vi "SubVI_SVM_gridsearch_n_fold.vi"(0 "Max Passes":i32=15, 5 "Training Labels":dbl[][](array[numeric]), 7 "Training Data":dbl[][](array[numeric]), 9 "Array":string[](array[string]), 10 "Optimizer\nMetric":string="F1", 11 "C":dbl[](array[numeric]), 12 "Gamma":dbl[](array[numeric])) -> (1 "Performance":T2, 2 "Hyperparameters":T1, 4 "Kernel Type":string, 6 "Alpha (idx)":dbl[][](array[numeric]), 8 "w":dbl[][](array[numeric]), 13 "label (idx)":dbl[][](array[numeric]), 14 "Training (idx)":dbl[][](array[numeric]), 15 "b":dbl)   [LabVIEW 2020]
uses:
  <vilib>/Analysis/baseanly.llb/Mean (DBL).vi
  <vilib>/Analysis/1siggen.llb/Riffle Array (DBL).vi
  <vilib>/Analysis/NI_AALBase.lvlib
panel:
  out "Numeric 3":i32
  out "Numeric 2":i32
  out "Numeric":i32
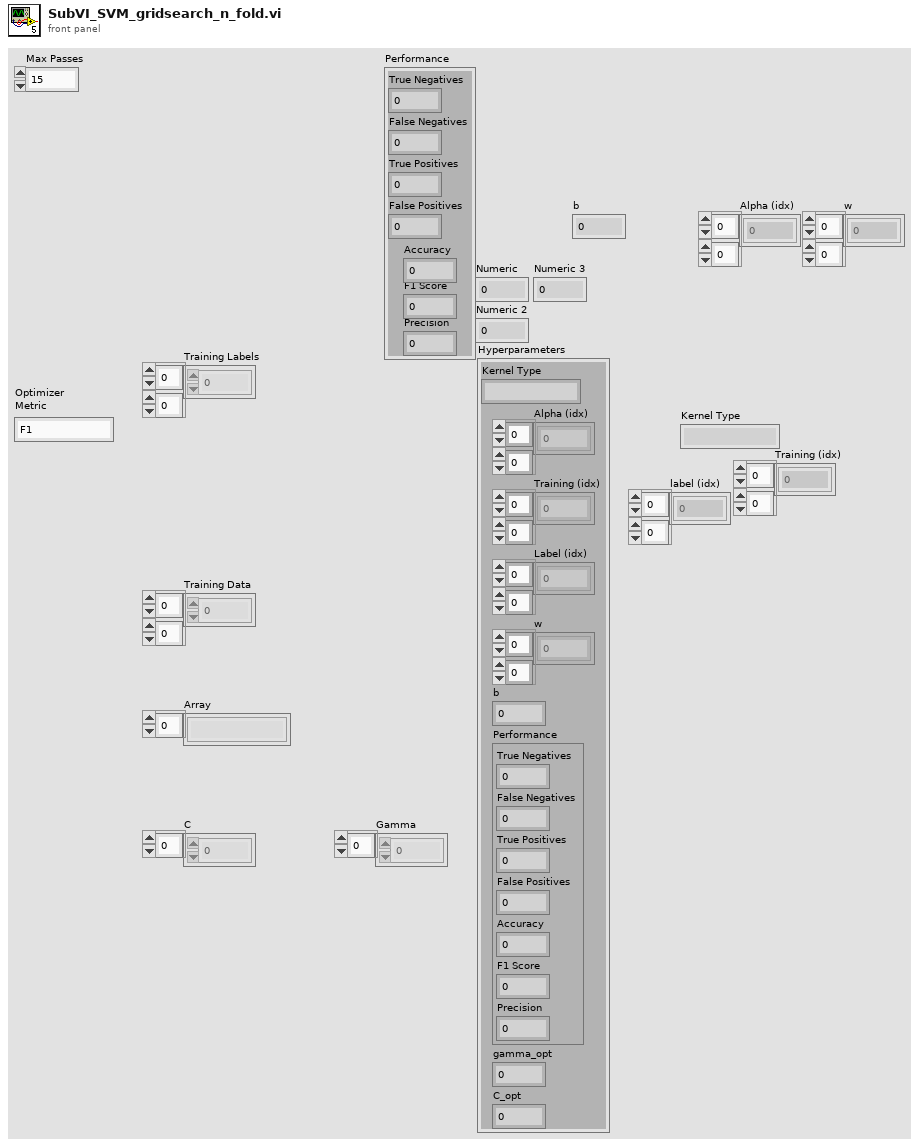
[diagram p1: front panel]
types:
  T1 = cluster{"Kernel Type":string, "Alpha (idx)":dbl[][], "Training (idx)":dbl[][], "Label (idx)":dbl[][], "w":dbl[][], "b":dbl, "Performance":cluster{"True Negatives":i32, "False Negatives":i32, "True Positives":i32, "False Positives":i32, "Accuracy":dbl, "F1 Score":dbl, "Precision":dbl}, "gamma_opt":dbl, "C_opt":dbl}
  T2 = cluster{"True Negatives":i32, "False Negatives":i32, "True Positives":i32, "False Positives":i32, "Accuracy":dbl, "F1 Score":dbl, "Precision":dbl}
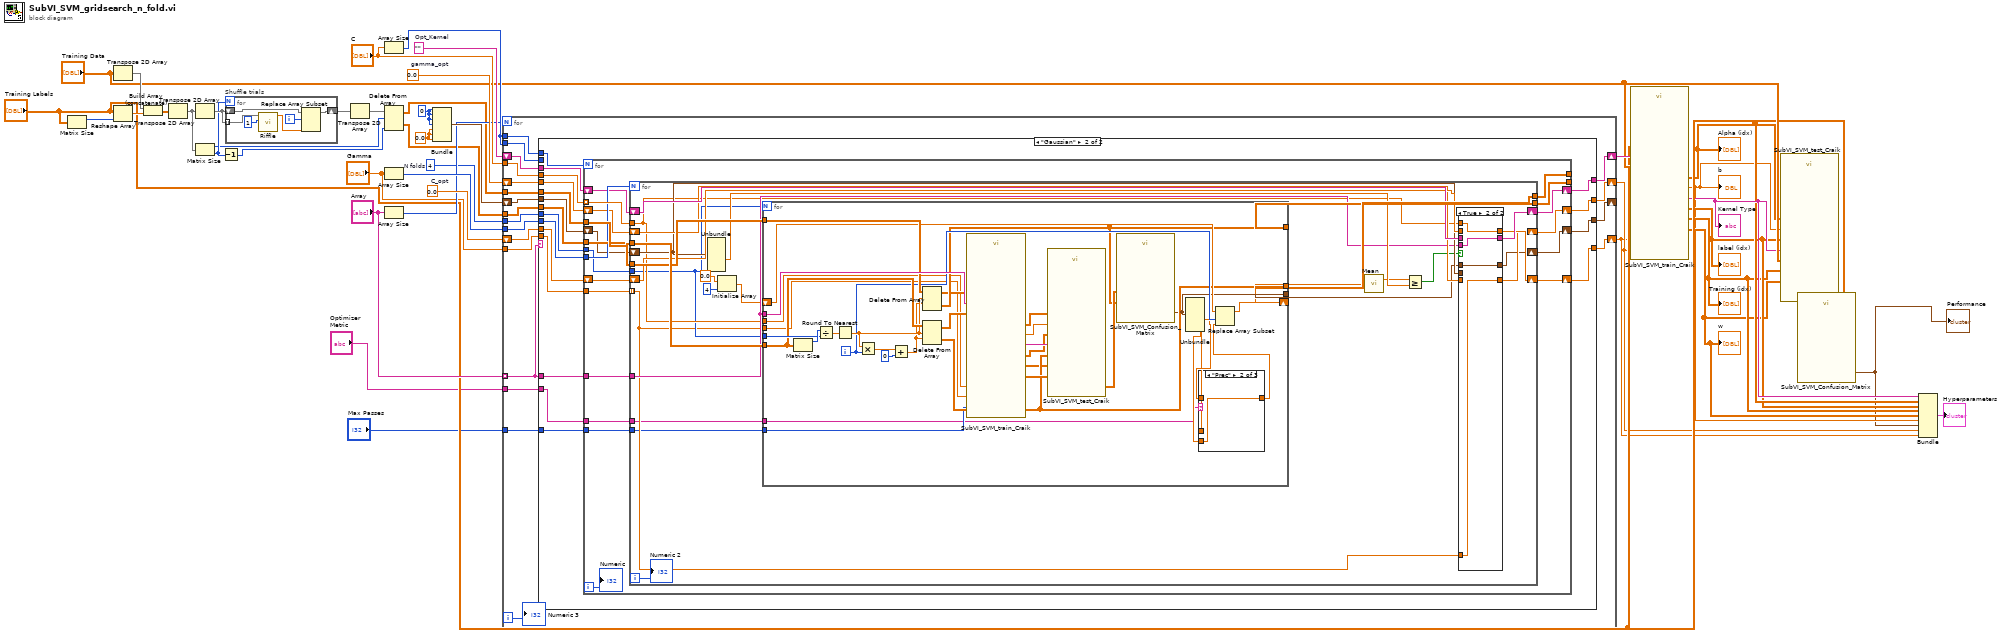
[diagram p0: block diagram]
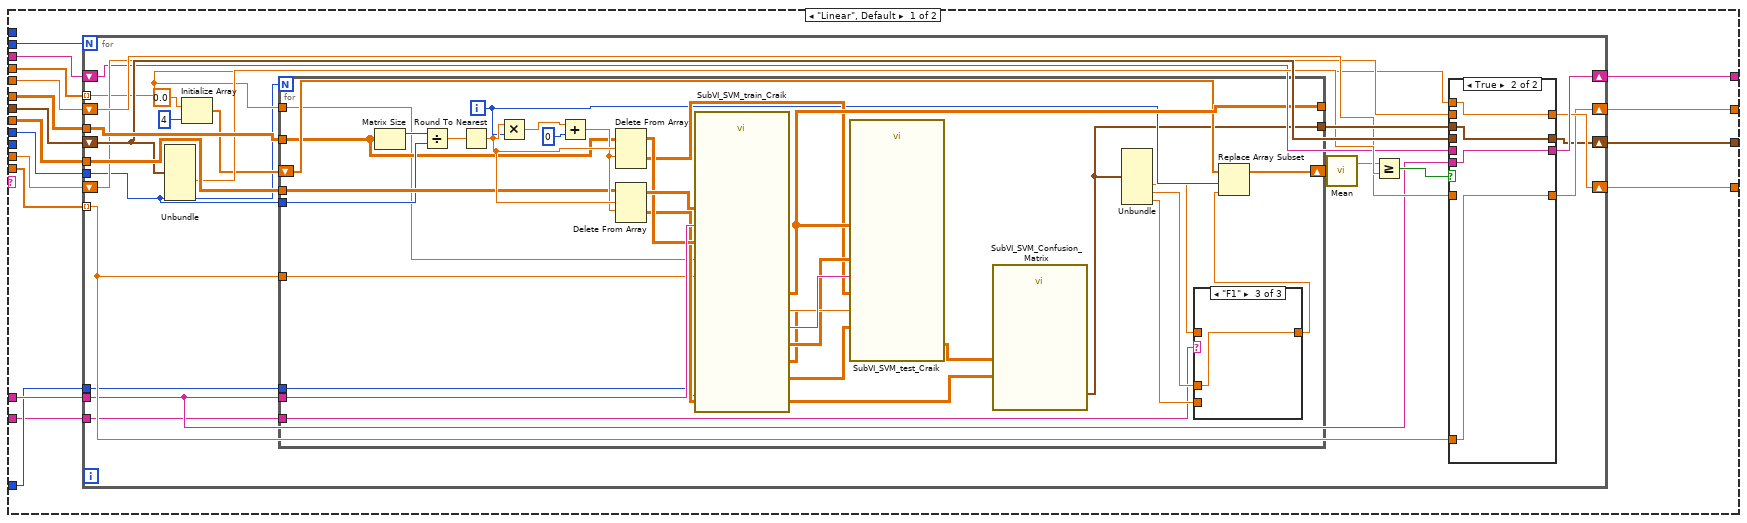
[diagram p2: hidden frame]
diagram:
  w32 = 4  # N folds
  w3 = 0.0
  w38 = 0
  w35 = ""  # Opt_Kernel
  w37 = 0.0  # gamma_opt
  w36 = 0.0  # C_opt
  n1 = Matrix Size(0:"Training Labels") -> (1:w29:i32)  [unwired: 1 out]
  n2 = Transpose 2D Array(2D array="Training Data") -> (transposed array=w28:dbl[][])
  n3 = Reshape Array("Training Labels", w29) -> (w31:dbl[])
  n4 = Build Array (concatenate)(w28, w31) -> (w30:dbl[][])
  n5 = Transpose 2D Array(2D array=w30) -> (transposed array=w21:dbl[][])
  n6 = Transpose 2D Array(2D array=w21) -> (transposed array=w27:dbl[][])
  n7 = Matrix Size(0:w21) -> (1:w23:i32, 2:w24:i32)
  n8 = Decrement(x=w24) -> (x-1=w22:i32)
  n9 = for "Shuffle trials" {
    N: w24 -> [_]
    tunnel: w27 -> [w48] mode=indexing
    shift-right: [w43] -> w26
    shift-left: w27 -> [w46]
    i -> [w44]
    n10 = call-poly <vilib>:"Riffle.vi"("seed"=1, "X"=w48) -> ("Riffled {X}"=w45:dbl[])  [unwired: 7 in, 2 out]
    n11 = Replace Array Subset(array=w46, new element=w45, index (row)=w44) -> (w43:dbl[][])  [unwired: 1 in]
  }
  n12 = Transpose 2D Array(2D array=w26) -> (transposed array=w25:dbl[][])
  n13 = Array Size(array="C") -> (size(s)=w40:i32)
  n14 = Delete From Array(array=w25, length=w23, index (col)=w22) -> (deleted portion=w19:dbl[][], array with subset deleted=w20:dbl[][])  [unwired: 1 in]
  n15 = Array Size(array="Gamma") -> (size(s)=w41:i32)
  n16 = Array Size(array="Array") -> (size(s)=w34:i32)
  n17 = Bundle(w38, w38, w38, w38, w3, w3, w3) -> (w39:cluster{i32, i32, i32, i32, dbl, dbl, dbl})  [unwired: 1 in]
  n18 = for {
    N: w34 -> [_]
    tunnel: "C" -> [w68]
    tunnel: "Array" -> [w64] mode=indexing
    tunnel: w20 -> [w67]
    tunnel: w19 -> [w66]
    tunnel: "Gamma" -> [w65]
    tunnel: w40 -> [w63]
    shift-right: [w61] -> w18
    shift-left: w35 -> [w62]
    shift-right: [w59] -> w6
    shift-left: w36 -> [w60]
    shift-right: [w57] -> w7
    shift-left: w37 -> [w58]
    shift-right: [w55] -> _
    shift-left: w39 -> [w56]
    tunnel: w40 -> [w54]
    tunnel: w41 -> [w53]
    tunnel: w32 -> [w52]
    tunnel: "Max Passes" -> [w50]
    tunnel: "Optimizer\nMetric" -> [w49]
    i -> [w51]
    n19 = case shown="\"Gaussian\"" w64 {
      tunnel: w68 -> [w85 w171]
      tunnel: w64 -> [w84 w170]
      tunnel: w67 -> [w83 w169]
      tunnel: w66 -> [w82 w168]
      tunnel: w65 -> [w81 w157]
      tunnel: w63 -> [w80 _]
      tunnel: w62 -> [w79 w165]
      tunnel: [w78 w158] -> w61
      tunnel: w60 -> [w77 w164]
      tunnel: [w76 w159] -> w59
      tunnel: w58 -> [w75 w163]
      tunnel: [w74 w160] -> w57
      tunnel: w56 -> [w73 w162]
      tunnel: [w72 w161] -> w55
      tunnel: w54 -> [_ w167]
      tunnel: w53 -> [_ w166]
      tunnel: w52 -> [w71 w156]
      tunnel: w50 -> [w70 w155]
      tunnel: w49 -> [w69 w154]
      frame "Linear", Default {
        n20 = for {
          N: w80 -> [_]
          tunnel: w85 -> [w94] mode=indexing
          tunnel: w84 -> [w99]
          tunnel: w83 -> [w109]
          tunnel: w82 -> [w108]
          tunnel: w81 -> [w102] mode=indexing
          shift-right: [w98] -> w78
          shift-left: w79 -> [w100]
          shift-right: [w97] -> w76
          shift-left: w77 -> [w101]
          shift-right: [w96] -> w74
          shift-left: w75 -> [w103]
          shift-right: [w95] -> w72
          shift-left: w73 -> [w107]
          tunnel: w71 -> [w88]
          tunnel: w70 -> [w87]
          tunnel: w69 -> [w86]
          n21 = Unbundle(w107) -> (w105:dbl)  [unwired: 6 out]
          n22 = Initialize Array(0.0 ("element"), 4 ("dimension size")) -> (w91:dbl[])
          n23 = for {
            N: w88 -> [_]
            tunnel: w109 -> [w119]
            tunnel: w108 -> [w128]
            tunnel: [w138] -> _
            tunnel: [w115] -> w106
            tunnel: w102 -> [w118]
            tunnel: w99 -> [w135]
            tunnel: w94 -> [w117]
            shift-right: [w121] -> w90
            shift-left: w91 -> [w123]
            tunnel: w88 -> [w120]
            tunnel: w87 -> [w116]
            tunnel: w86 -> [w110]
            i -> [w122]
            n24 = Matrix Size(0:w119) -> (1:w134:i32)  [unwired: 1 out]
            n25 = Divide(x=w134, y=w120) -> (x/y=w133:dbl)
            n26 = Round To Nearest(number=w133) -> (nearest integer value=w130:dbl)
            n27 = Multiply(x=w130, y=w122) -> (x*y=w131:dbl)
            n28 = Add(x=w131, y=0) -> (x+y=w129:dbl)
            n29 = Delete From Array(array=w119, length=w130, index (row)=w129) -> (deleted portion=w125:dbl[][], array with subset deleted=w126:dbl[][])  [unwired: 1 in]
            n30 = Delete From Array(array=w128, length=w130, index (row)=w129) -> (deleted portion=w124:dbl[][], array with subset deleted=w127:dbl[][])  [unwired: 1 in]
            n31 = call "SubVI_SVM_train_Craik.vi"("Max Passes"=w116, "C"=w117, "Label Data"=w127, "Gamma"=w118, "Linear or Gaussian"=w135, "Training Data"=w126) -> ("Alpha (idx)"=w138:dbl[][], "Label (idx)"=w136:dbl[][], "b"=w139:dbl, "Training (idx)"=w137:dbl[][], "w"=w140:dbl[][], "Kernel Type"=w141:string)
            n32 = call "SubVI_SVM_test_Craik.vi"("Alpha (idx)"=w138, "Testing Data"=w125, "Label (idx)"=w136, "training (idx)"=w137, "Linear or Gaussian"=w141, "b"=w139, "w"=w140) -> ("Prediction"=w142:dbl[][])  [unwired: 4 in]
            n33 = call "SubVI_SVM_Confusion_Matrix.vi"("Real Labels"=w124, "Predictions"=w142) -> ("Performance"=w115:T2)  [unwired: 9 in]
            n34 = Unbundle(w115) -> ("Accuracy"=w112:dbl, "F1 Score"=w113:dbl, "Precision"=w114:dbl)  [unwired: 4 out]
            n35 = case shown="\"F1\"" w110 {
              tunnel: w114 -> [_ w144 _]
              tunnel: w113 -> [_ _ w145]
              tunnel: w112 -> [w143 _ _]
              tunnel: [w143 w144 w145] -> w111
              frame "Acc", Default {
              }
              frame "Prec" {
              }
              frame "F1" {
              }
            }
            n36 = Replace Array Subset(array=w123, new element=w111, index=w122) -> (w121:dbl[])
          }
          n37 = call-poly <vilib>:"Mean.vi"("X"=w90) -> ("mean"=w89:dbl)  [unwired: 1 out]
          n38 = Greater Or Equal?(x=w89, y=w105) -> (x >= y?=w104:bool)
          n39 = case shown="True" w104 {
            tunnel: w107 -> [w146 _]
            tunnel: w106 -> [_ w150]
            tunnel: w103 -> [w147 _]
            tunnel: w102 -> [_ w151]
            tunnel: w94 -> [_ w152]
            tunnel: w101 -> [w148 _]
            tunnel: w100 -> [w149 _]
            tunnel: w99 -> [_ w153]
            tunnel: [w149 w153] -> w98
            tunnel: [w148 w152] -> w97
            tunnel: [w147 w151] -> w96
            tunnel: [w146 w150] -> w95
            frame False {
            }
            frame True {
            }
          }
        }
      }
      frame "Gaussian" {
        n40 = for {
          N: w167 -> [_]
          tunnel: w171 -> [w191] mode=indexing
          tunnel: [w190] -> _
          tunnel: [w189] -> _
          tunnel: w170 -> [w188]
          tunnel: w169 -> [w187]
          tunnel: w168 -> [w186]
          tunnel: w157 -> [w185]
          tunnel: w166 -> [w184]
          shift-right: [w179] -> w158
          shift-left: w165 -> [w183]
          shift-right: [w178] -> w159
          shift-left: w164 -> [w182]
          shift-right: [w177] -> w160
          shift-left: w163 -> [w181]
          shift-right: [w176] -> w161
          shift-left: w162 -> [w180]
          tunnel: w156 -> [w175]
          tunnel: w155 -> [w173]
          tunnel: w154 -> [w172]
          i -> [w174]
          n41 = for {
            N: w184 -> [_]
            tunnel: w191 -> [w207]
            tunnel: [w218] -> w190
            tunnel: [w217] -> w189
            tunnel: w188 -> [w208]
            tunnel: w187 -> [w216]
            tunnel: w186 -> [w215]
            tunnel: w185 -> [w196] mode=indexing
            shift-right: [w205] -> w179
            shift-left: w183 -> [w214]
            shift-right: [w204] -> w178
            shift-left: w182 -> [w213]
            shift-right: [w203] -> w177
            shift-left: w181 -> [w212]
            shift-right: [w193] -> w176
            shift-left: w180 -> [w210]
            tunnel: w175 -> [w202]
            tunnel: w173 -> [w194]
            tunnel: w172 -> [w192]
            i -> [w195]
            n42 = Unbundle(w210) -> (w211:dbl)  [unwired: 6 out]
            n43 = Initialize Array(0.0 ("element"), 4 ("dimension size")) -> (w199:dbl[])
            n44 = for {
              N: w202 -> [_]
              tunnel: [w231] -> w218
              tunnel: [w233] -> w217
              tunnel: w216 -> [w240]
              tunnel: w215 -> [w239]
              tunnel: w208 -> [w249]
              tunnel: w207 -> [w228]
              tunnel: w196 -> [w229]
              tunnel: [w224] -> w206
              tunnel: w202 -> [w244]
              shift-right: [w234] -> w198
              shift-left: w199 -> [w236]
              tunnel: w194 -> [w225]
              tunnel: w192 -> [w219]
              i -> [w235]
              n45 = Matrix Size(0:w240) -> (1:w245:i32)  [unwired: 1 out]
              n46 = Divide(x=w245, y=w244) -> (x/y=w243:dbl)
              n47 = Round To Nearest(number=w243) -> (nearest integer value=w238:dbl)
              n48 = Multiply(x=w238, y=w235) -> (x*y=w241:dbl)
              n49 = Add(x=w241, y=0) -> (x+y=w237:dbl)
              n50 = Delete From Array(array=w239, length=w238, index (row)=w237) -> (deleted portion=w233:dbl[][], array with subset deleted=w232:dbl[][])  [unwired: 1 in]
              n51 = Delete From Array(array=w240, length=w238, index (row)=w237) -> (deleted portion=w231:dbl[][], array with subset deleted=w230:dbl[][])  [unwired: 1 in]
              n52 = call "SubVI_SVM_train_Craik.vi"("Max Passes"=w225, "C"=w228, "Label Data"=w232, "Gamma"=w229, "Linear or Gaussian"=w249, "Training Data"=w230) -> ("Alpha (idx)"=w248:dbl[][], "Label (idx)"=w227:dbl[][], "b"=w247:dbl, "Training (idx)"=w226:dbl[][], "w"=w246:dbl[][], "Kernel Type"=w250:string)
              n53 = call "SubVI_SVM_test_Craik.vi"("Alpha (idx)"=w248, "Testing Data"=w231, "Label (idx)"=w227, "training (idx)"=w226, "Linear or Gaussian"=w250, "b"=w247, "w"=w246) -> ("Prediction"=w251:dbl[][])  [unwired: 4 in]
              n54 = call "SubVI_SVM_Confusion_Matrix.vi"("Real Labels"=w233, "Predictions"=w251) -> ("Performance"=w224:T2)  [unwired: 9 in]
              n55 = Unbundle(w224) -> ("Accuracy"=w223:dbl, "F1 Score"=w222:dbl, "Precision"=w221:dbl)  [unwired: 4 out]
              n56 = case shown="\"Prec\"" w219 {
                tunnel: w221 -> [_ w253 _]
                tunnel: w222 -> [_ _ w254]
                tunnel: w223 -> [w252 _ _]
                tunnel: [w252 w253 w254] -> w220
                frame "Acc", Default {
                }
                frame "Prec" {
                }
                frame "F1" {
                }
              }
              n57 = Replace Array Subset(array=w236, new element=w220, index=w235) -> (w234:dbl[])
            }
            n58 = call-poly <vilib>:"Mean.vi"("X"=w198) -> ("mean"=w197:dbl)  [unwired: 1 out]
            n59 = Greater Or Equal?(x=w197, y=w211) -> (x >= y?=w209:bool)
            n60 = case shown="True" w209 {
              tunnel: w214 -> [w258 _]
              tunnel: w213 -> [w257 _]
              tunnel: w212 -> [w256 _]
              tunnel: w210 -> [w255 _]
              tunnel: w208 -> [_ w262]
              tunnel: w207 -> [_ w261]
              tunnel: w196 -> [_ w260]
              tunnel: w206 -> [_ w259]
              tunnel: [w258 w262] -> w205
              tunnel: [w257 w261] -> w204
              tunnel: [w256 w260] -> w203
              tunnel: [w255 w259] -> w193
              frame False {
              }
              frame True {
              }
            }
            "Numeric 2" <- w195
          }
          "Numeric" <- w174
        }
      }
    }
    "Numeric 3" <- w51
  }
  n61 = call "SubVI_SVM_train_Craik.vi"("C"=w6, "Label Data"="Training Labels", "Gamma"=w7, "Linear or Gaussian"=w18, "Training Data"="Training Data") -> ("Alpha (idx)"=w12:dbl[][], "Label (idx)"=w10:dbl[][], "b"=w8:dbl, "Training (idx)"=w11:dbl[][], "w"=w9:dbl[][], "Kernel Type"=w13:string)  [unwired: 1 in]
  "Alpha (idx)" <- w12
  "b" <- w8
  "label (idx)" <- w11
  "Kernel Type" <- w13
  "Training (idx)" <- w10
  "w" <- w9
  n62 = call "SubVI_SVM_test_Craik.vi"("Alpha (idx)"=w12, "Testing Data"="Training Data", "Label (idx)"=w10, "training (idx)"=w11, "Linear or Gaussian"=w13, "b"=w8, "w"=w9) -> ("Prediction"=w16:dbl[][])  [unwired: 4 in]
  n63 = call "SubVI_SVM_Confusion_Matrix.vi"("Real Labels"="Training Labels", "Predictions"=w16) -> ("Performance"=w4:T2)  [unwired: 9 in]
  "Performance" <- w4
  n64 = Bundle("Kernel Type"=w13, "Alpha (idx)"=w12, "Training (idx)"=w11, "Label (idx)"=w10, "w"=w9, "b"=w8, "Performance"=w4, "gamma_opt"=w7, "C_opt"=w6) -> (→"Hyperparameters":T1)  [unwired: 1 in]
